vi "Utility Firmware Info.vi"(5 "Retry Attempts (0)":i32 min=0, 7 "Fast Comms (F)":bool, 8 "error in":errorcluster, 11 "VISA resource name":refnum<visa-resource-name>) -> (0 "error out":errorcluster, 1 "Firmware Version":string, 2 "Firmware Part Number":dbl, 3 "VISA resource name out":refnum<visa-resource-name>)   [LabVIEW 2020, in "ChromTech Series I Drivers.lvlib"]
doc: "Returns the firmware version and part number. For Series I, the part number is not returned and will always be zero."
uses:
  <instrlib>/RxnRover/ChromtechSeriesIDriver/ChromTech Series I Drivers.lvlib
panel:
  out "Response":string
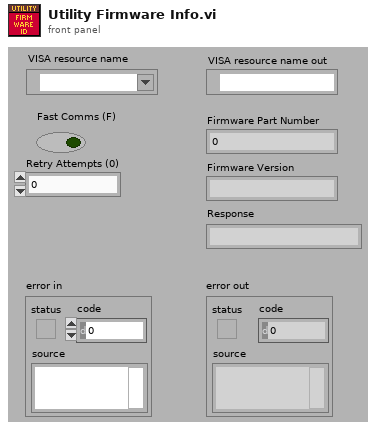
[diagram p1: front panel]
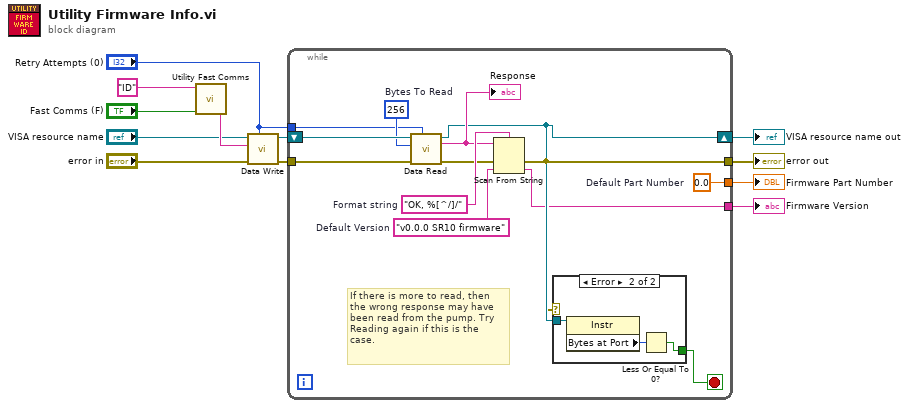
[diagram p0: block diagram]
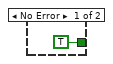
[diagram p2: hidden frame]
diagram:
  n1 = call <instrlib>:"Utility Fast Comms.vi"("Fast Comms"="Fast Comms (F)", "Command"="ID") -> ("Fast Command"=w11:string)  [unwired: 9 in]
  n2 = call <instrlib>:"Data Write.vi"("Retry Attempts (0)"="Retry Attempts (0)", "error in (no error)"="error in", "Command"=w11, "VISA Refnum in"="VISA resource name") -> ("error out"=w7:errorcluster, "VISA Refnum out"=w6:refnum<visa-resource-name>)  [unwired: 6 in]
  n3 = while {
    tunnel: [w15] -> w9
    tunnel: [w13] -> w8
    tunnel: "Retry Attempts (0)" -> [w19]
    shift-right: [w18] -> w2
    shift-left: w6 -> [w22]
    tunnel: w7 -> [w23]
    tunnel: [w17] -> w1
    stop <- w16 stop-if-true
    w21 = u32 256  # Bytes To Read
    w14 = "v0.0.0 SR10 firmware"  # Default Version
    w15 = 0.0  # Default Part Number
    w25 = "OK, %[^/]/"  # Format string
    # "If there is more to read, then\nthe wrong response may have\nbeen read from the pump. Try\nReading again if this is the\ncase."
    n4 = call <instrlib>:"Data Read.vi"("Retry Attempts (0)"=w19, "error in (no error)"=w23, "Bytes to read"=w21, "VISA Refnum in"=w22) -> ("error out"=w24:errorcluster, "read buffer"=w20:string, "VISA Refnum out"=w18:refnum<visa-resource-name>)  [unwired: 5 in]
    "Response" <- w20
    n5 = Scan From String(format string=w25, input string=w20, error in=w24, default 1=w14) -> (error out=w17:errorcluster, output 1=w13:string)  [unwired: 1 in, 2 out]
    n6 = case shown="Error" w17 {
      tunnel: w18 -> [_ w29]
      tunnel: [TRUE w27] -> w16
      frame No Error {
      }
      frame Error {
        n7 = property class="Instr"(reference=w29) -> ("Bytes at Port"=w28:u32)  [unwired: 1 in, 2 out]
        n8 = Less Or Equal To 0?(x=w28) -> (x <= 0?=w27:bool)
      }
    }
  }
  "VISA resource name out" <- w2
  "error out" <- w1
  "Firmware Part Number" <- w9
  "Firmware Version" <- w8
